vi "allpaths.vi"(0 "Array":path[](array[path])) -> ()   [LabVIEW 2010]
panel:
  # "help"
  # "curr"
  # "home"
  # "default data"
  # "lib"
  # "app"
  # "temp"
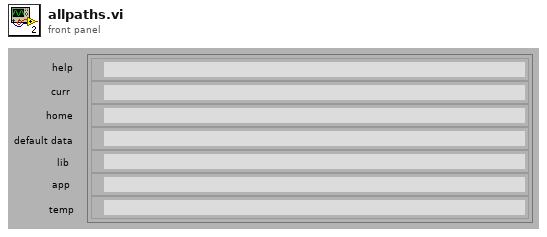
[diagram p1: front panel]
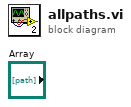
[diagram p0: block diagram]
diagram:
